vi "noRepaetFileName(SubVI).vi"(3 "ext":string, 4 "file name":string="abc", 5 "subID":string="sub-00", 6 "directory Path":path) -> (0 "file path out":path)   [LabVIEW 2021]
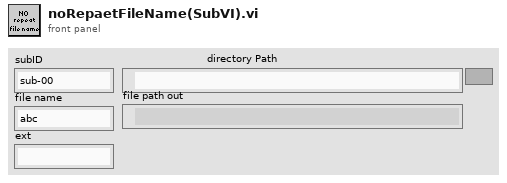
[diagram p1: front panel]
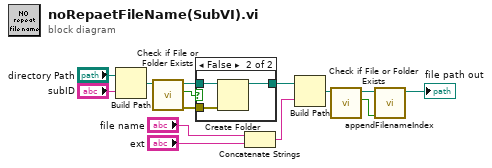
[diagram p0: block diagram]
diagram:
  n1 = Build Path(base path="directory Path", name or relative path="subID") -> (appended path=w10:path)
  n2 = call <vilib>:"Check if File or Folder Exists.vi"("path"=w10) -> ("error out"=w12:errorcluster, "file or folder exists?"=w9:bool, "dup path"=w11:path)  [unwired: 8 in]
  n3 = case shown="False" w9 {
    tunnel: [w15 w18] -> w5
    tunnel: w11 -> [w15 w17]
    tunnel: w12 -> [_ w16]
    frame True {
    }
    frame False {
      n4 = Create Folder(path (use dialog)=w17, error in=w16) -> (created path=w18:path)  [unwired: 1 in, 2 out]
    }
  }
  n5 = Concatenate Strings("file name", "ext") -> (w13:string)
  n6 = Build Path(base path=w5, name or relative path=w13) -> (appended path=w7:path)
  n7 = call <vilib>:"Check if File or Folder Exists.vi"("path"=w7) -> ("file or folder exists?"=w1:bool, "dup path"=w2:path)  [unwired: 8 in, 1 out]
  n8 = call "appendFilenameIndex.vi"("newFile? (no:F)"=w1, "dup path"=w2) -> ("appended path"=→"file path out":path)  [unwired: 9 in]
